vi "Create_data_log_file.vi"(8 "error in (no error)":errorcluster, 10 "Export Folder Path":path, 11 "Byte Stream File in":refnum<file>) -> (0 "error out":errorcluster, 3 "Byte Stream File out":refnum<file>)   [LabVIEW 2013]
doc: "Creates a log file if not created already, only if reference is empty"
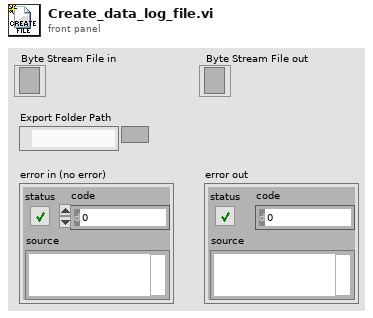
[diagram p1: front panel]
types:
  T1 = enum16{"open", "replace", "create", "open or create", "replace or create", "replace or create with confirmation"}
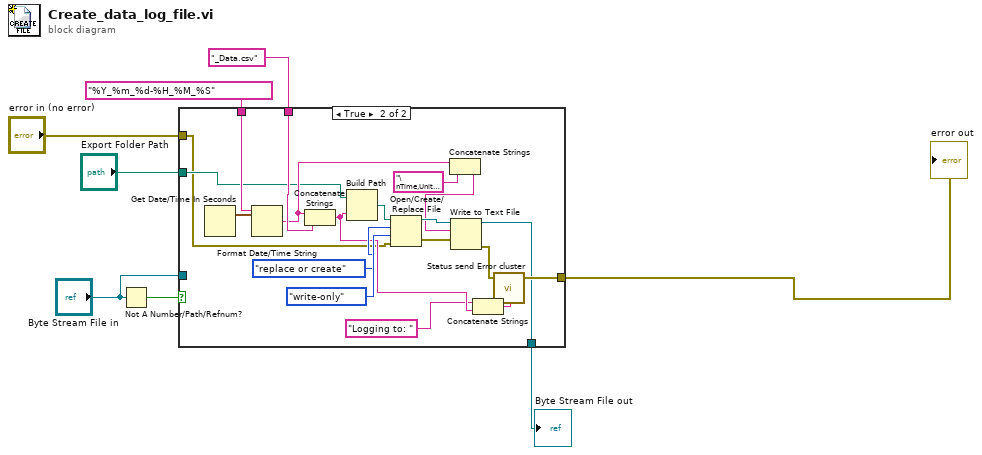
[diagram p0: block diagram]
diagram:
  n1 = Not A Number/Path/Refnum?(number/path/refnum="Byte Stream File in") -> (NaN/Path/Refnum?=w6:bool)
  n2 = case shown="True" w6 {
    tunnel: "_Data.csv" ("name or relative path") -> [_ w19]
    tunnel: "%Y_%m_%d-%H_%M_%S" -> [_ w17]
    tunnel: "Export Folder Path" -> [_ w14]
    tunnel: "error in (no error)" -> [w10 w13]
    tunnel: [w10 w12] -> w5
    tunnel: [w9 w11] -> w7
    tunnel: "Byte Stream File in" -> [w9 _]
    frame False {
      # "file alteady created, do not create another"
    }
    frame True {
      n3 = Get Date/Time In Seconds() -> (seconds since 1Jan1904=w29:timestamp)
      n4 = Format Date/Time String(time format string (%c)=w17, seconds (now)=w29) -> (date/time string=w15:string)  [unwired: 1 in]
      n5 = Concatenate Strings(w15, w19) -> (w21:string)
      n6 = Build Path(base path=w14, name or relative path=w21) -> (appended path=w25:path)
      n7 = Open/Create/Replace File(file path (use dialog)=w25, error in=w13, operation (0:open)=T1."replace or create", access (0:read/write)=enum16{"read/write", "read-only", "write-only"}."write-only") -> (refnum out=w24:refnum<file>, error out=w28:errorcluster)  [unwired: 2 in, 1 out]
      n8 = Concatenate Strings(w15, "\nTime,Unit,Sample#,sens.type1,val1,...\n" ("text")) -> (w16:string)
      n9 = Write to Text File(file (use dialog)=w24, text=w16, error in=w28) -> (refnum out=w11:refnum<file>, error out=w23:errorcluster)  [unwired: 1 in, 1 out]
      n10 = Concatenate Strings("Logging to: " ("string"), w21) -> (w22:string)
      n11 = call "Status send Error cluster.vi"("error in (no error)"=w23, "Send status msg \"XXX\" or don't wire for no message"=w22) -> ("error out"=w12:errorcluster)  [unwired: 7 in]
    }
  }
  "Byte Stream File out" <- w7
  "error out" <- w5
